vi "Pop Chart (Triple).vi"(0 "Waveform Chart":refnum<vi>) -> ()   [LabVIEW 2013]
panel:
  in  "Close Chart":bool
  out "Waveform Chart":dbl[][](graph)
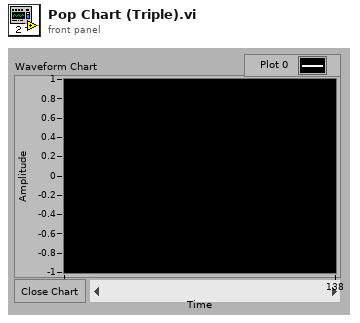
[diagram p1: front panel]
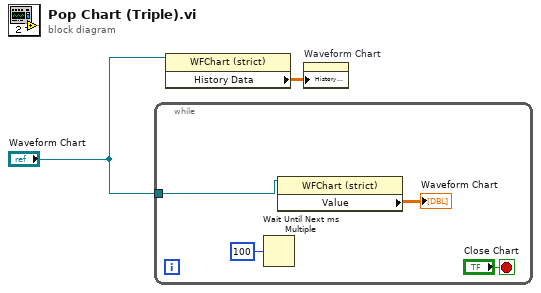
[diagram p0: block diagram]
diagram:
  n1 = while {
    tunnel: "Waveform Chart" -> [w3]
    stop <- "Close Chart" stop-if-true
    n2 = Wait Until Next ms Multiple(millisecond multiple=u32 100) -> ()  [unwired: 1 out]
    n3 = property class="WFChart (strict)"(reference=w3) -> ("Value"=→"Waveform Chart":dbl[][])  [unwired: 1 in, 2 out]
  }
  n4 = property class="WFChart (strict)"(reference="Waveform Chart") -> ("History Data"=w2:dbl[][])  [unwired: 1 in, 2 out]
  n5 = property on="Waveform Chart" class="WFChart (strict)"("History Data"=w2) -> ()  [unwired: 2 in, 2 out]
